vi "ds_Reflection Point.vi"(0 "points before":dbl[][](array[numeric]) format="%.2f", 1 "function and data":T1, 3 "high index":u32=1, 5 "psum before":dbl[](array[numeric]) format="%.2f", 9 "f values before":dbl[](array[numeric]) format="%.2f", 11 "error in (no error)":errorcluster, 12 "factor":dbl format="%.2f") -> (4 "points after":dbl[][](array[numeric]) format="%.2f", 6 "psum after":dbl[](array[numeric]) format="%.2f", 8 "number of function calls":i32, 10 "f values after":dbl[](array[numeric]) format="%.2f", 14 "new f value":dbl format="%.2f", 15 "error out":errorcluster)   [LabVIEW 2020, in "NI_Gmath.lvlib"]
uses:
  <vilib>/gmath/NI_Gmath.lvlib
  <vilib>/gmath/NumericalOptimization/ucno_user function ref and data.ctl
  <vilib>/gmath/NumericalOptimization/ucno_user objective function ref.ctl
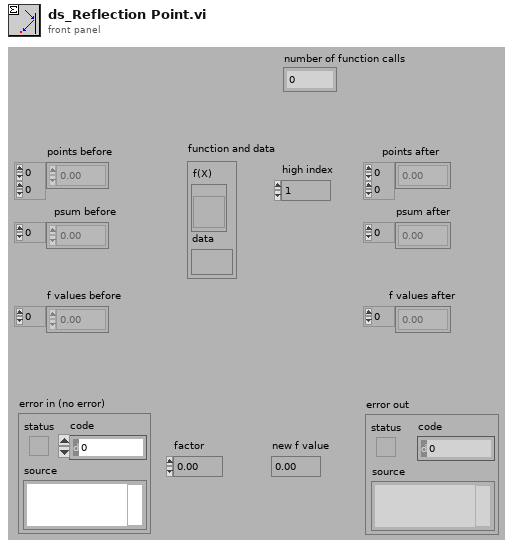
[diagram p1: front panel]
types:
  T1 = typedef "NI_Gmath.lvlib/ucno_user function ref and data.ctl" = cluster{"f(X)":T2, "data":variant}
  T2 = typedef "NI_Gmath.lvlib/ucno_user objective function ref.ctl" = refnum<vi>
  T3 = cluster{"objective function":bool, "gradient":bool}
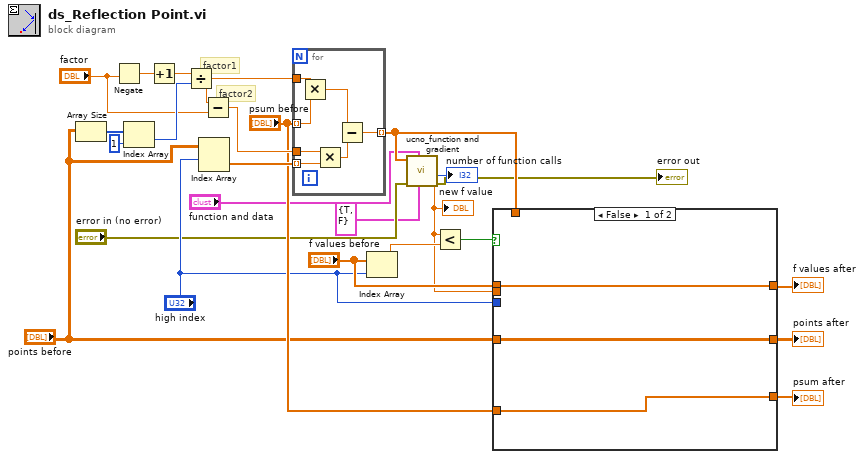
[diagram p0: block diagram]
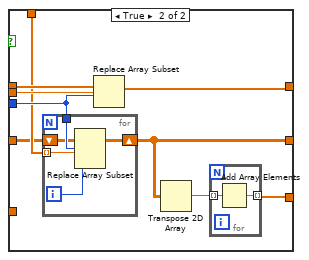
[diagram p2: hidden frame]
diagram:
  # "factor2"
  # "factor1"
  n1 = Array Size(array="points before") -> (size(s)=w25:i32[])
  n2 = Negate(x="factor") -> (-x=w23:dbl)
  n3 = Index Array(array=w25, index=1) -> (element=w21:i32)
  n4 = Increment(x=w23) -> (x+1=w22:dbl)
  n5 = Divide(x=w22, y=w21) -> (x/y=w20:dbl)
  n6 = Index Array(array="points before", index (row)="high index") -> (element=w18:dbl[])  [unwired: 1 in]
  n7 = Subtract(x=w20, y="factor") -> (x-y=w17:dbl)
  n8 = for {
    tunnel: w20 -> [w32]
    tunnel: "psum before" -> [w31] mode=indexing
    tunnel: w18 -> [w30] mode=indexing
    tunnel: w17 -> [w29]
    tunnel: [w26] -> w8 mode=indexing
    n9 = Multiply(x=w32, y=w31) -> (x*y=w28:dbl)
    n10 = Multiply(x=w29, y=w30) -> (x*y=w27:dbl)
    n11 = Subtract(x=w28, y=w27) -> (x-y=w26:dbl)
  }
  n12 = Index Array(array="f values before", index="high index") -> (element=w12:dbl)
  n13 = call <vilib>:"ucno_function and gradient.vi"("output control"=T3 {"objective function"=TRUE, "gradient"=FALSE}, "function and data"="function and data", "error in (no error)"="error in (no error)", "X"=w8) -> ("error out"=→"error out":errorcluster, "number of function calls"=→"number of function calls":i32, "f(X)"=w6:dbl)  [unwired: 4 in, 1 out]
  "new f value" <- w6
  n14 = Less?(x=w6, y=w12) -> (x < y?=w7:bool)
  n15 = case shown="False" w7 {
    tunnel: "psum before" -> [w35 _]
    tunnel: [w35 w38] -> w15
    tunnel: "points before" -> [w34 w37]
    tunnel: [w34 w36] -> w13
    tunnel: "f values before" -> [w33 w44]
    tunnel: [w33 w42] -> w10
    tunnel: "high index" -> [_ w41]
    tunnel: w6 -> [_ w43]
    tunnel: w8 -> [_ w40]
    frame False {
    }
    frame True {
      n16 = for {
        tunnel: w41 -> [w50]
        tunnel: w40 -> [w49] mode=indexing
        shift-right: [w47] -> w36
        shift-left: w37 -> [w48]
        i -> [w51]
        n17 = Replace Array Subset(array=w48, new element=w49, index (row)=w50, index (col)=w51) -> (w47:dbl[][])
      }
      n18 = Replace Array Subset(array=w44, new element=w43, index=w41) -> (w42:dbl[])
      n19 = Transpose 2D Array(2D array=w36) -> (transposed array=w39:dbl[][])
      n20 = for {
        tunnel: w39 -> [w46] mode=indexing
        tunnel: [w45] -> w38 mode=indexing
        n21 = Add Array Elements(numeric array=w46) -> (sum=w45:dbl)
      }
    }
  }
  "points after" <- w13
  "psum after" <- w15
  "f values after" <- w10
